vi "Set Up Buffers.vi"(4 "Output Data 2":variant, 6 "Output Data 1":variant, 8 "error in (no error)":errorcluster, 10 "Root Actor In":refnum<class "Root Actor.lvclass">, 11 "System Modules Factory in":refnum<class "System Modules Factory.lvclass">) -> (0 "error out":errorcluster, 2 "Root Actor Out":refnum<class "Root Actor.lvclass">, 3 "System Modules Factory out":refnum<class "System Modules Factory.lvclass">)   [LabVIEW 2019, in "System Modules Factory.lvclass"]
uses:
  System Modules Factory.lvclass
  Actor/Root Actor/Root Actor.lvclass
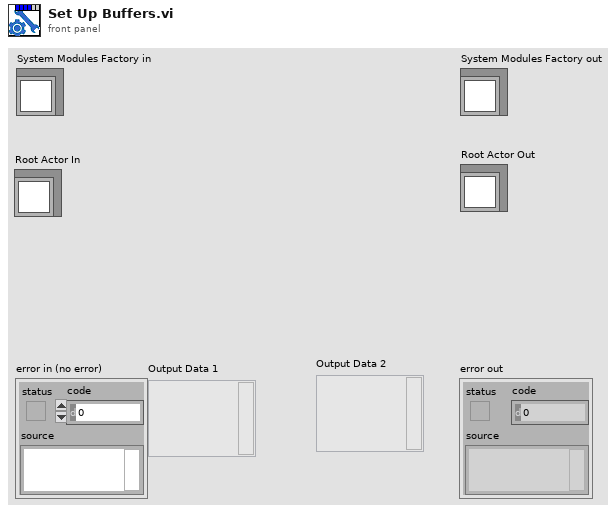
[diagram p1: front panel]
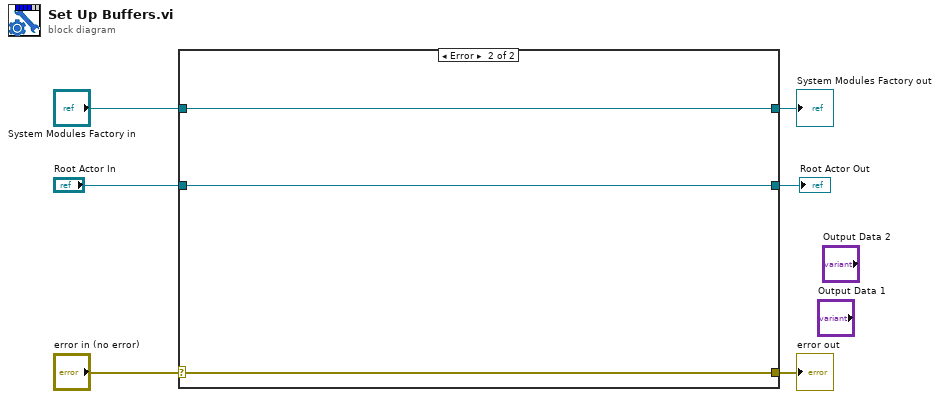
[diagram p0: block diagram]
diagram:
  n1 = case shown="Error" "error in (no error)" {
    selector: "error in (no error)" -> [w8 w12]
    tunnel: [w8 w12] -> w5
    tunnel: [w9 w11] -> w3
    tunnel: "System Modules Factory in" -> [w9 w11]
    tunnel: [w7 w10] -> w2
    tunnel: "Root Actor In" -> [w7 w10]
    frame No Error {
      # "Wire the error cluster across even in the \"No Error\"\ncase so that warnings get propagated."
    }
    frame Error {
    }
  }
  "error out" <- w5
  "System Modules Factory out" <- w3
  "Root Actor Out" <- w2
